vi "get device info from controls.vi"(8 "error in (no error)":errorcluster, 11 "Caller VI ref":refnum<vi>) -> (0 "error out":errorcluster, 3 "GUIDeviceInfo":T1)   [LabVIEW 2020]
uses:
  Device Driver/GUIDeviceInfo_TypDEf.ctl
  MySQL/Preset Query Enum.ctl
  <userlib>/_OpenG.lib/array/array.llb/Search 1D Array (String)__ogtk.vi
  <userlib>/_OpenG.lib/array/array.llb/Index 1D Array Elements (String)__ogtk.vi
panel:
  out "Array":string[](array[string])
  out "Array 3":string[](array[string])
  out "Caller variable names":string[](array[string])
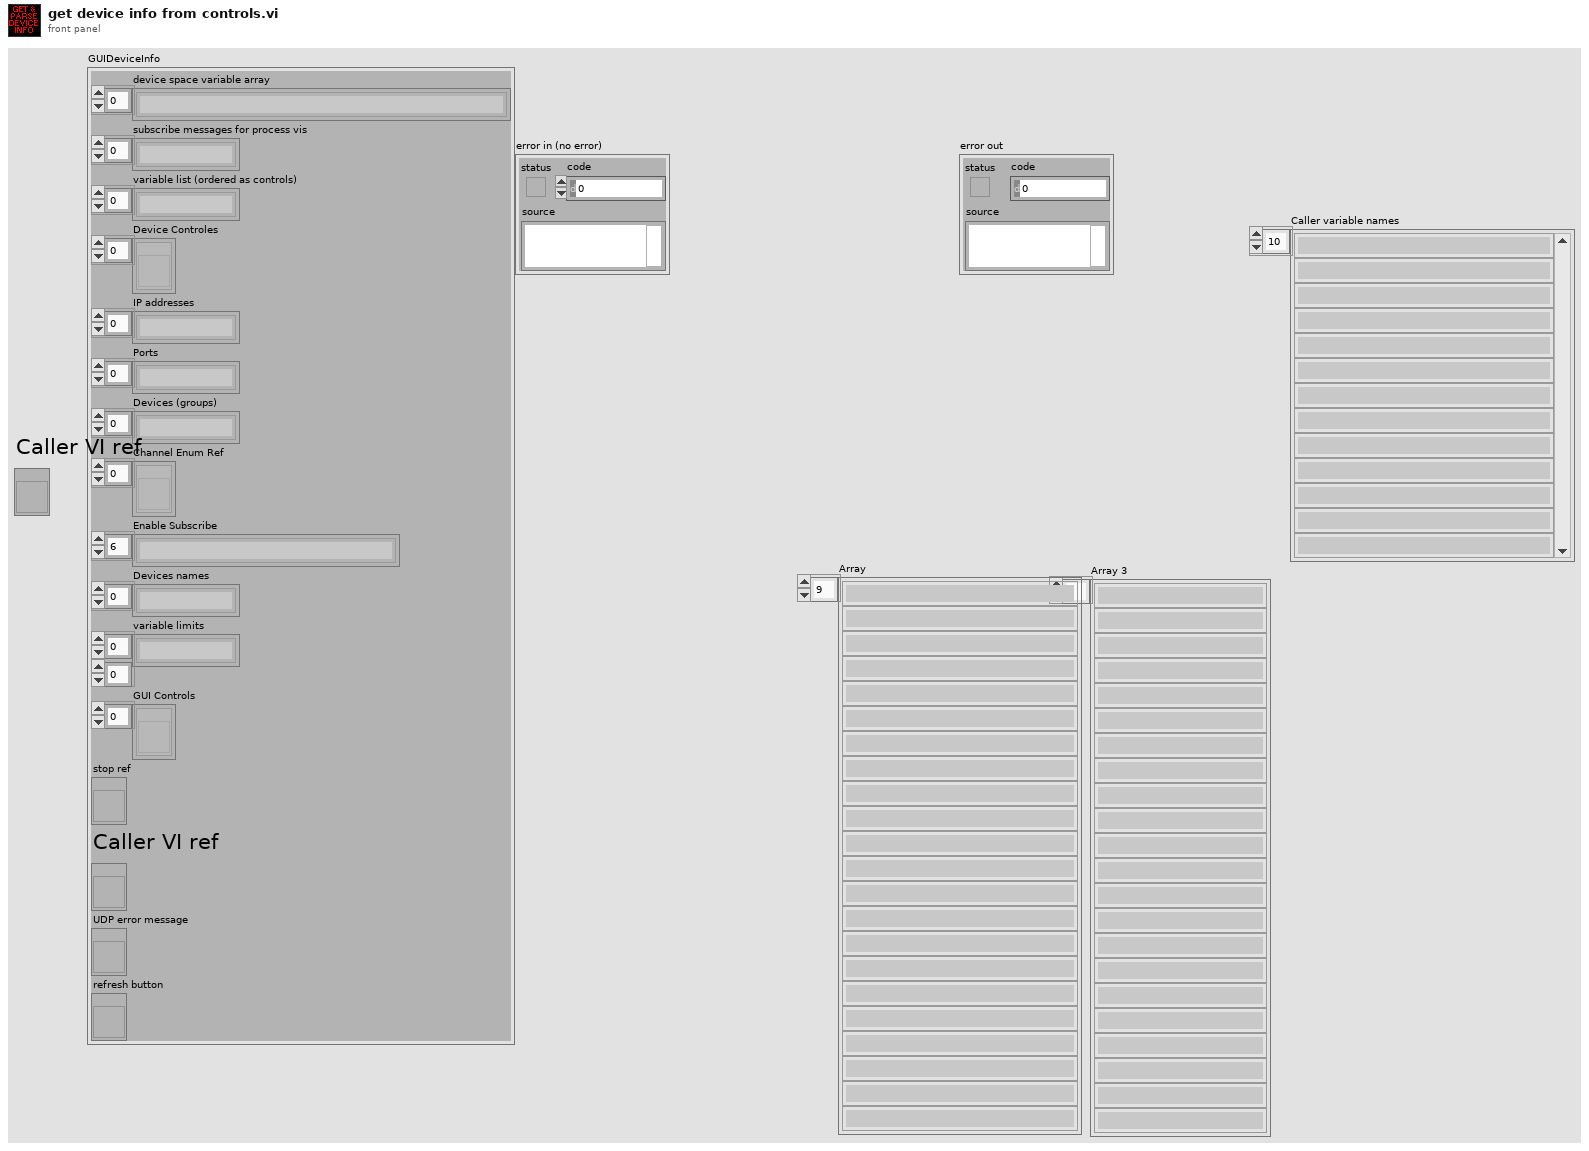
[diagram p1: front panel]
types:
  T1 = typedef "GUIDeviceInfo_TypDEf.ctl" = cluster{"device space variable array":string[], "subscribe messages for process vis":string[], "variable list (ordered as controls)":string[], "Device Controles":refnum<vi>[], "IP addresses":string[], "Ports":string[], "Devices (groups)":string[], "Channel Enum Ref":refnum<vi>[], "Enable Subscribe":string[], "Devices names":string[], "variable limits":string[][], "GUI Controls ":refnum<vi>[], "stop ref":refnum<vi>, "Caller VI ref":refnum<vi>, "UDP error message":refnum<vi>, "refresh button":refnum<vi>}
  T2 = typedef "Preset Query Enum.ctl" = enum16{"Get Locations", "Get all IPs and MACs", "Get classes", "Get expt variables to set at scanstart for particular device", "Get expt devices and variables with start values", "Get expt devices and variables (with data to get)", "Get expt devices with data to get", "Get Expt devices and GUIs", "Get all devices basic properties", "Get Virtual Devices Core Info", "Get Expt names", "Get experiment basic properties", "Get experiment alarm variables", "Get MC Ports", "Get device network comm port", "Get devicetype lvclass path", "Get basic device properties", "Get Init Order", "Get all setable variables of a device", "Get device variable aliases", "Get force values of all settable variables", "Get all variables of a devicetype", "Get all variables of a device", "Get plotter details", "Get Saved Scans", "Get Scan Info", "GetGeneralGUIs", "Get expt for plotter", "Get plotter IDs from expt", "Get all devices", "Get all Virtual Devices", "Get all aliases", "Get variable and device info for Virtual Device", "GetItemLocatorIP", "Get IPs for GUIs", "Get DeviceType from Device", "GetLocalPortRange", "GetDevicePresetVariables", "Get Device Configuration", "GetAllPresetNames", "GetAllConfigurationNames", "GetPresetDeviceNames", "GetDeviceAliases", "GetDevicesOfClass"}
  T3 = enum8{"Enabled", "Disabled", "Disabled and Grayed Out"}
  T4 = typedef "GUI_control_ref.ctl" = cluster{"UDP error message":refnum<vi>, "refresh button":refnum<vi>, "stop ref":refnum<vi>}
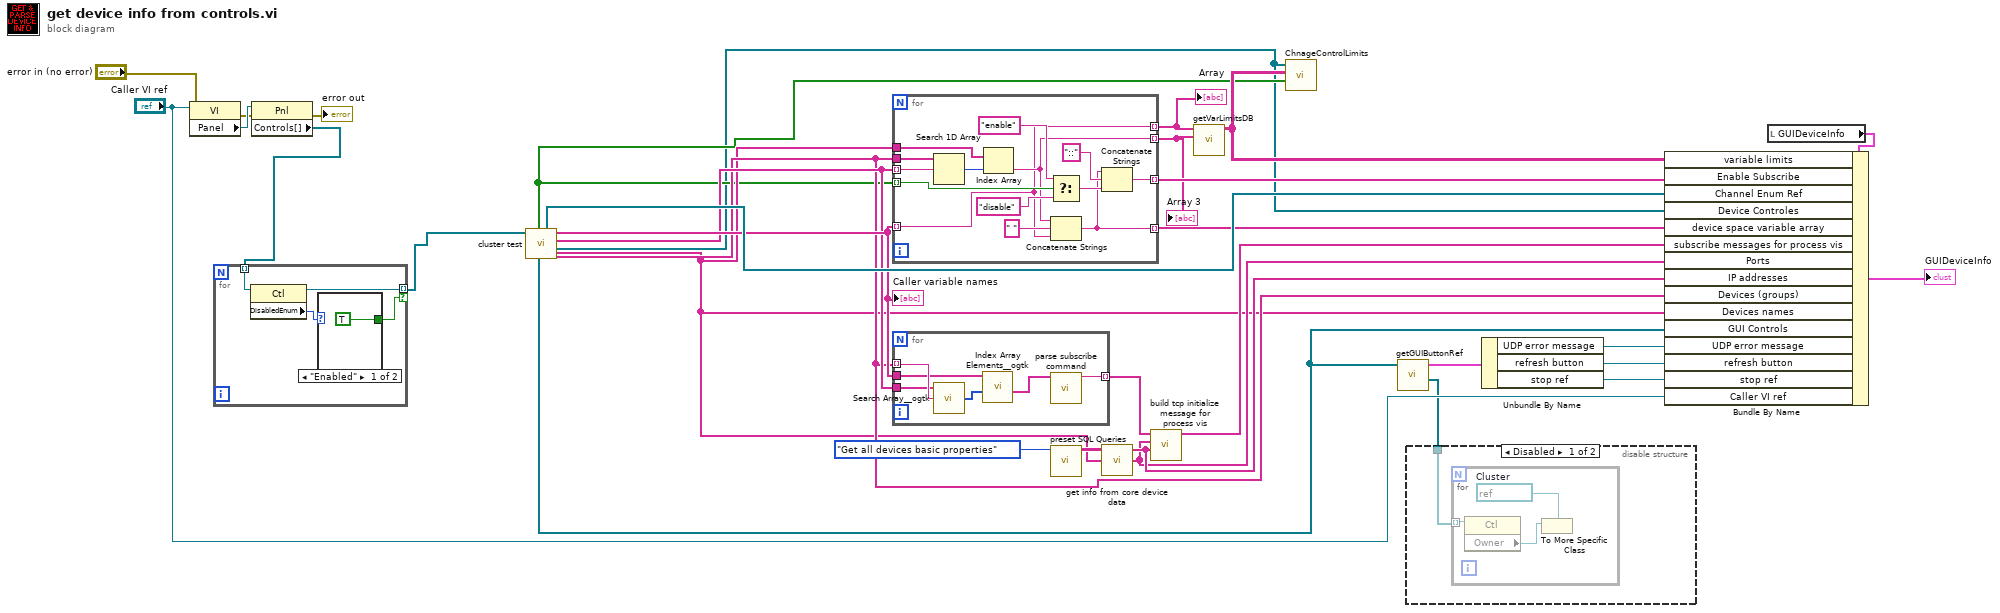
[diagram p0: block diagram]
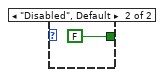
[diagram p2: hidden frame]
diagram:
  n1 = property class="VI"(reference="Caller VI ref", error in="error in (no error)") -> (error out=w14:errorcluster, "Panel"=w15:refnum<vi>)  [unwired: 1 out]
  n2 = property class="Pnl"(reference=w15, error in=w14) -> (error out=→"error out":errorcluster, "Controls[]"=w2:refnum<vi>[])  [unwired: 1 out]
  n3 = for {
    tunnel: w2 -> [w37] mode=indexing
    tunnel: [w35] -> w1 mode=indexing if=w34
    n4 = property class="Ctl"(reference=w37) -> (reference out=w35:refnum<vi>, "DisabledEnum"=w36:T3)  [unwired: 1 in, 1 out]
    n5 = case shown="\"Enabled\"" w36 {
      tunnel: [TRUE FALSE] -> w34
      frame "Enabled" {
      }
      frame "Disabled", Default {
      }
    }
  }
  n6 = call "cluster test.vi"("Controls[]"=w1) -> ("Dev groups (numbers)"=w20:string[], "Device controles"=w3:refnum<vi>[], "variable dev numbers"=w21:string[], "Caller variable names"=w22:string[], "Device Names"=w19:string[], "Enum controls"=w25:refnum<vi>[], "GUI Controls"=w10:refnum<vi>[], "Enable Subscribe"=w11:bool[])  [unwired: 3 in]
  "Caller variable names" <- w22
  n7 = for {
    tunnel: w22 -> [w40] mode=indexing
    tunnel: w21 -> [w52] mode=indexing
    tunnel: w20 -> [w53]
    tunnel: w19 -> [w51]
    tunnel: [w43] -> w24 mode=indexing
    tunnel: w11 -> [w47] mode=indexing
    tunnel: [w42] -> w23 mode=indexing
    tunnel: [w41] -> w17 mode=indexing
    tunnel: [w40] -> w18 mode=indexing
    n8 = Search 1D Array(1D array=w53, element=w52) -> (index of element=w49:i32)  [unwired: 1 in]
    n9 = Index Array(array=w51, index=w49) -> (element=w41:string)
    n10 = Select(t="enable" ("f"), s=w47, f="disable") -> (s? t:f=w44:string)
    n11 = Concatenate Strings(w41, " " ("string"), w40) -> (w43:string)
    n12 = Concatenate Strings(w43, "::" ("string"), w44) -> (w42:string)
  }
  "Array 3" <- w17
  "Array" <- w18
  n13 = for {
    tunnel: w20 -> [w59] mode=indexing
    tunnel: w21 -> [w57]
    tunnel: [w55] -> w26 mode=indexing
    tunnel: w22 -> [w54]
    n14 = call-poly <userlib>:"Search Array__ogtk.vi"("Array"=w57, "Element Data"=w59) -> ("Indices of Elements"=w58:i32[])  [unwired: 7 in]
    n15 = call-poly <userlib>:"Index Array Elements__ogtk.vi"("indices"=w58, "array"=w54) -> ("elements"=w56:string[])  [unwired: 9 in]
    n16 = call "parse subscribe command.vi"("variable names"=w56) -> ("Subscribe command"=w55:string)  [unwired: 6 in]
  }
  n17 = call "preset SQL Queries.vi"("Preset Query"=Preset_Query_Enum."Get all devices basic properties") -> ("data"=w29:string[][])  [unwired: 8 in, 2 out]
  n18 = call "get info from core device data.vi"("devices to get data from"=w19, "All Devices Core Info"=w29) -> ("Ports"=w31:string[], "IP Addresses"=w32:string[])  [unwired: 2 in]
  n19 = call "build tcp initialize message for process vis.vi"("IP Addresses"=w32, "Ports"=w31, "Subscribe commands"=w26) -> ("subscribe messages\nfor process vis"=w30:string[])  [unwired: 8 in]
  n20 = call "getVarLimitsDB.vi"("devices in"=w17, "variables in"=w18) -> ("limits out"=w16:string[][])  [unwired: 9 in]
  n21 = call "ChnageControlLimits.vi"("Enable Subscribe"=w11, "limits out"=w16, "Control references"=w3) -> ()  [unwired: 9 in]
  n22 = call "getGUIButtonRef.vi"("Controls[]"=w10) -> ("channelSelectro ref"=w4:refnum<vi>[], "button ref out"=w9:T4)  [unwired: 9 in]
  n23 = disable-structure shown="Disabled" {
    disable-tunnel: w4 -> [w60 _]
    frame Disabled {
      n24 = for {
        tunnel: w60 -> [w63] mode=indexing
        w61 = refnum<vi> refnum  # Cluster
        n25 = property class="Ctl"(reference=w63) -> ("Owner"=w62:refnum<vi>)  [unwired: 1 in, 2 out]
        n26 = To More Specific Class(target class=w61, reference=w62) -> ()  [unwired: 1 in, 2 out]
      }
    }
    frame Enabled {
    }
  }
  n27 = Unbundle By Name(w9) -> ("UDP error message"=w8:refnum<vi>, "refresh button"=w7:refnum<vi>, "stop ref"=w6:refnum<vi>)
  n28 = local read "GUIDeviceInfo"() -> (w27:T1)
  n29 = Bundle By Name(cluster=w27, "variable limits"=w16, "Enable Subscribe"=w23, "Channel Enum Ref"=w25, "Device Controles"=w3, "device space variable array"=w24, "subscribe messages for process vis"=w30, "Ports"=w31, "IP addresses"=w32, "Devices (groups)"=w20, "Devices names"=w19, "GUI Controls"=w10, "UDP error message"=w8, "refresh button"=w7, "stop ref"=w6, "Caller VI ref"="Caller VI ref") -> (→"GUIDeviceInfo":T1)
